vi "ChangeConfigServer.vi"(4 "error in (no error)":errorcluster) -> (0 "error out":errorcluster)   [LabVIEW 2015]
doc: "This GUI interprets supplied configuration information and displays it to the user. It compares the target configuration to the machine state (what components are loaded) and checks for compatibility. If the user choses to start a move, an enumerated script is output that can be used to start a sequence of moves."
uses:
  Script_actions.ctl
  Utils/ChangeConfig.ctl
  Users/Sherman/Desktop/BETA_GSCS/Systems/SystemUtil/Command.ctl
  Users/Sherman/Desktop/BETA_GSCS/GUI/GSP_GUI_global.vi
  TCPServer/TCP_Global.vi
panel:
  out "First Attempt to change?":bool
  out "Used setup Cmd":bool
  in  "Configuration":i32(listbox)
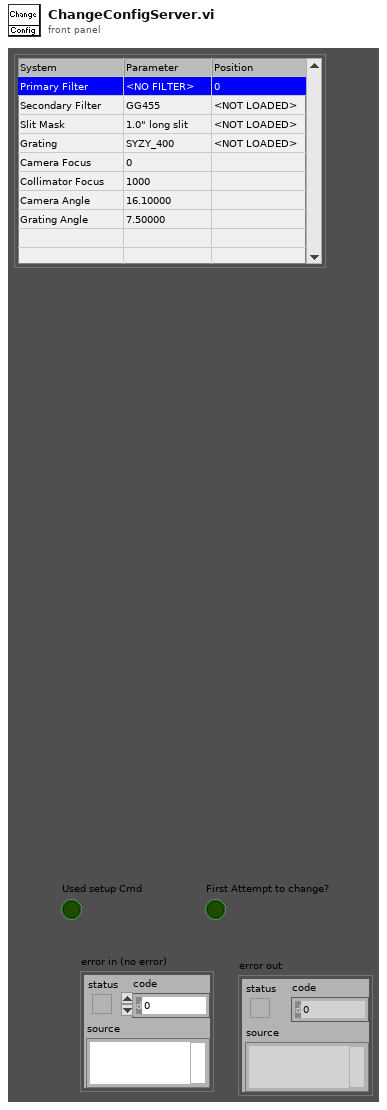
[diagram p1: front panel]
types:
  T1 = typedef "Command.ctl" = cluster{"Command":string, "Parameter":string}
  T2 = typedef "ChangeConfig.ctl" = cluster{"Command":string, "Configuration":cluster{"Primary Filter":string, "Secondary Filter":string, "Slit Mask":string, "Grating":string, "CS Target":dbl, "GS Target":dbl, "Coll Focus":i32, "Camera Focus":i32, "use Flexure Comp?":bool, "WavMode":string, "Slit Toggle":string}}
  T3 = cluster{"Primary Filter Slot":i32, "Secondary Filter Slot":i32, "Slit#":i32, "Grating#":i32, "CS Angle":dbl, "GS Angle":dbl, "Coll Focus":i32, "Camera Focus":i32, "Select Mode":i32, "Flexure":bool, "Slit Toggle":bool}
  T4 = typedef "Script_actions.ctl" = enum16{"Change Primary Filter", "Change Secondary Filter", "Change Collimator Focus", "Change Camera Focus", "Change Grating", "Change Angles", "Change Slit Mask", "Toggle Slit", "Change WAVMODE", "Check All Systems", "Change Flexure"}
  T5 = cluster{"Grating#":i32, "Slit#":i32, "Primary Filter#":i32, "Secondary Filter#":i32, "Coll Position":i32, "Camera Focus":i32, "Camera Angle":dbl, "Grating Angle":dbl, "Coll Temp":dbl, "CF Temp\n":dbl, "Camera Target":dbl, "Grating Target":dbl, "WAVMODE":string, "Slit Hidden??":bool}
  T6 = cluster{"Primary Filter":string, "Secondary Filter":string, "Slit Mask":string, "Grating":string, "CS Target":dbl, "GS Target":dbl, "Coll Focus":i32, "Camera Focus":i32, "use Flexure Comp?":bool, "WavMode":string, "Slit Toggle":string}
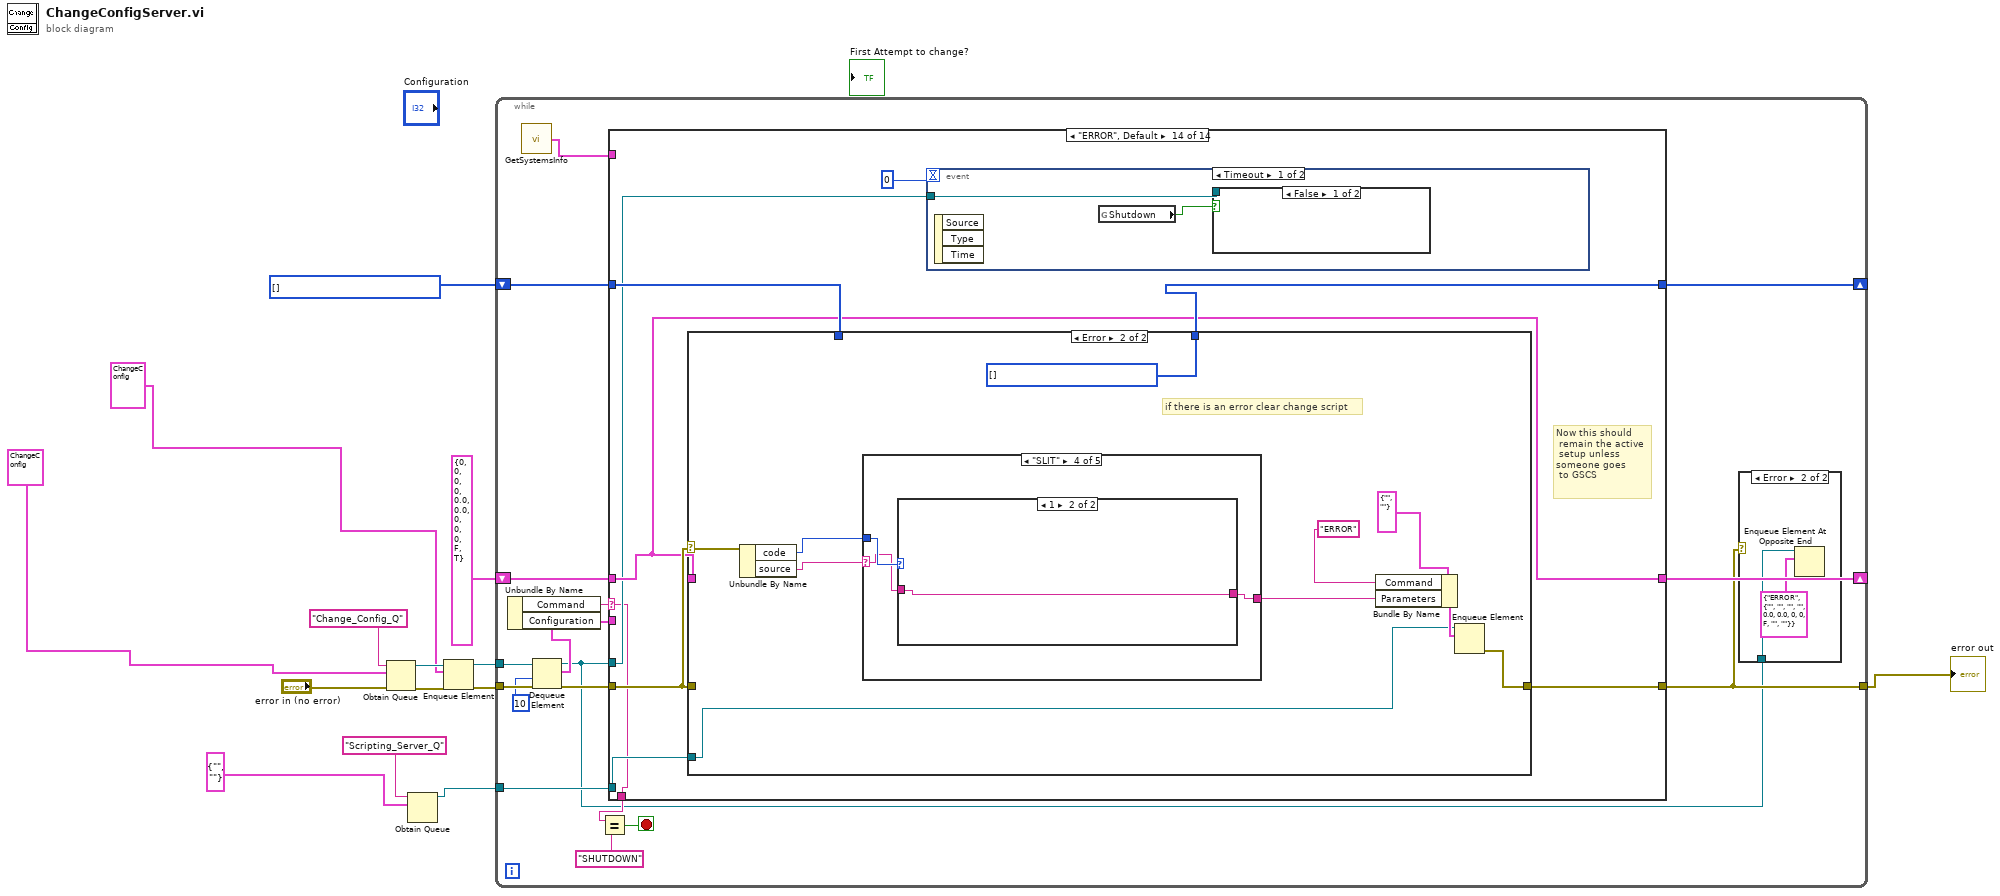
[diagram p0: block diagram]
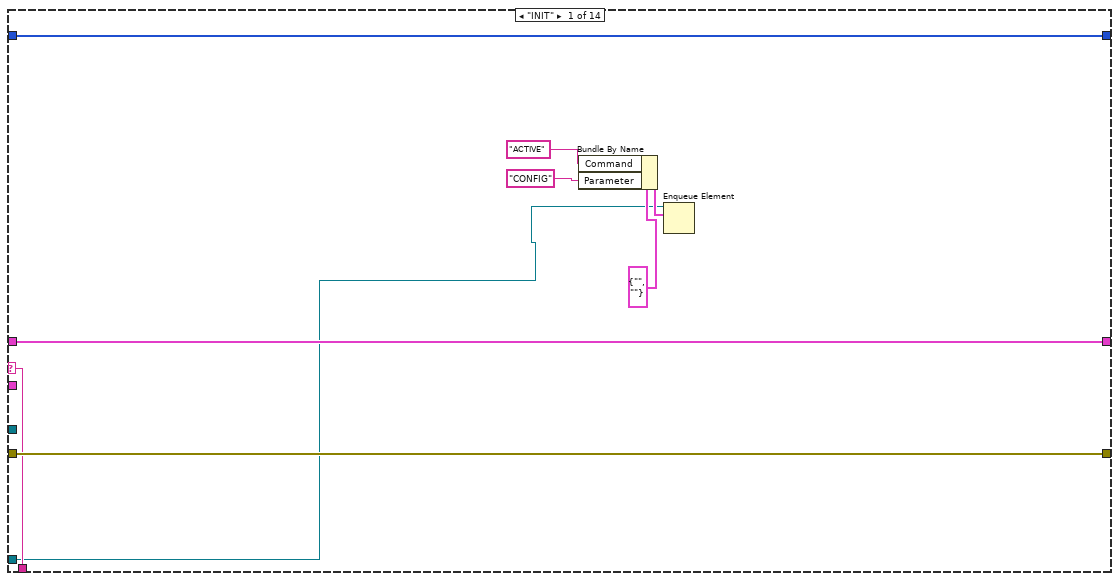
[diagram p3: hidden frame]
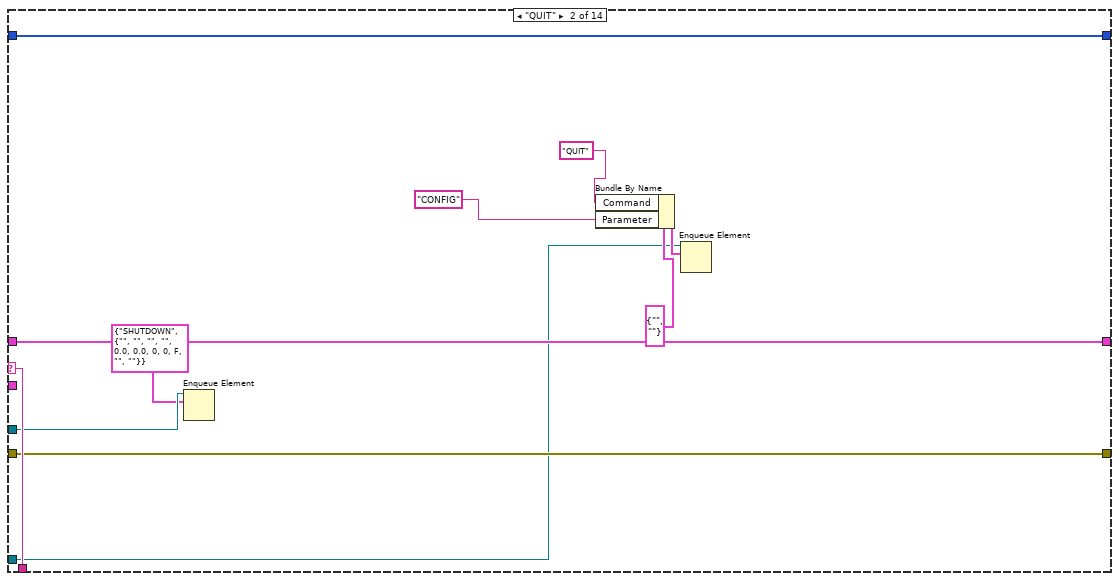
[diagram p4: hidden frame]
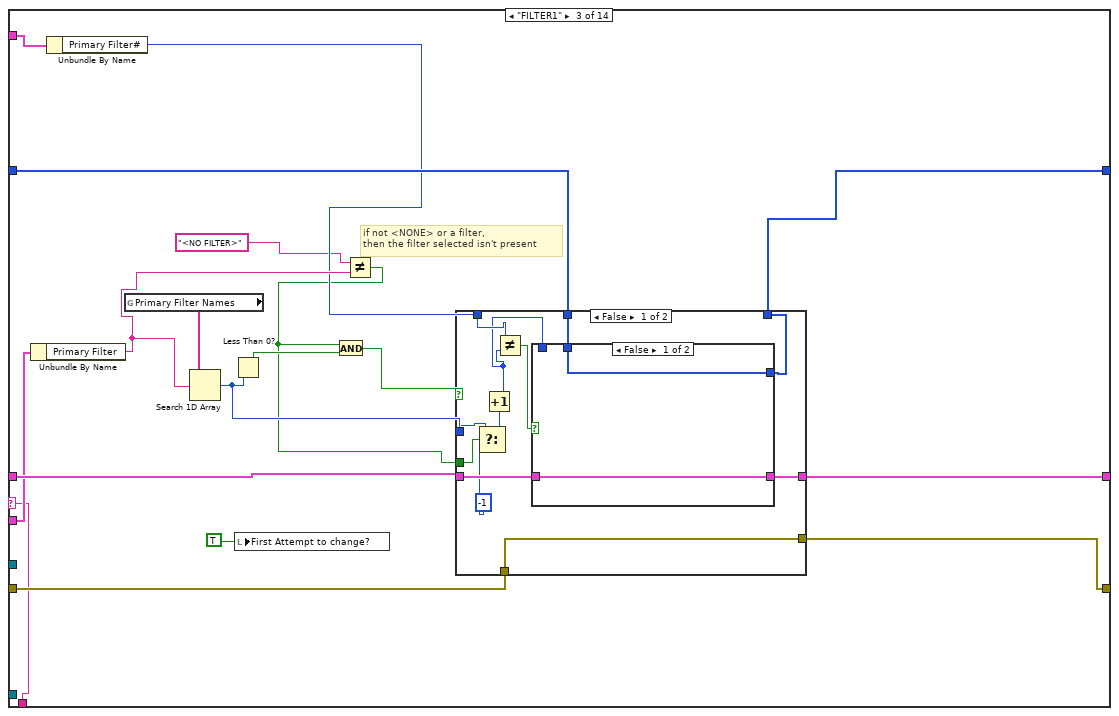
[diagram p5: hidden frame]
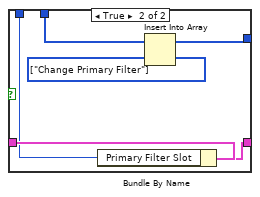
[diagram p6: hidden frame]
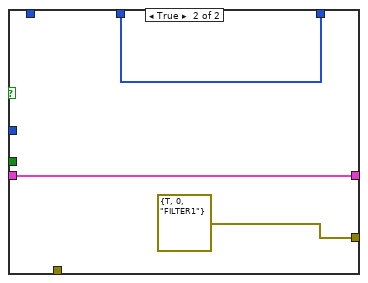
[diagram p7: hidden frame]
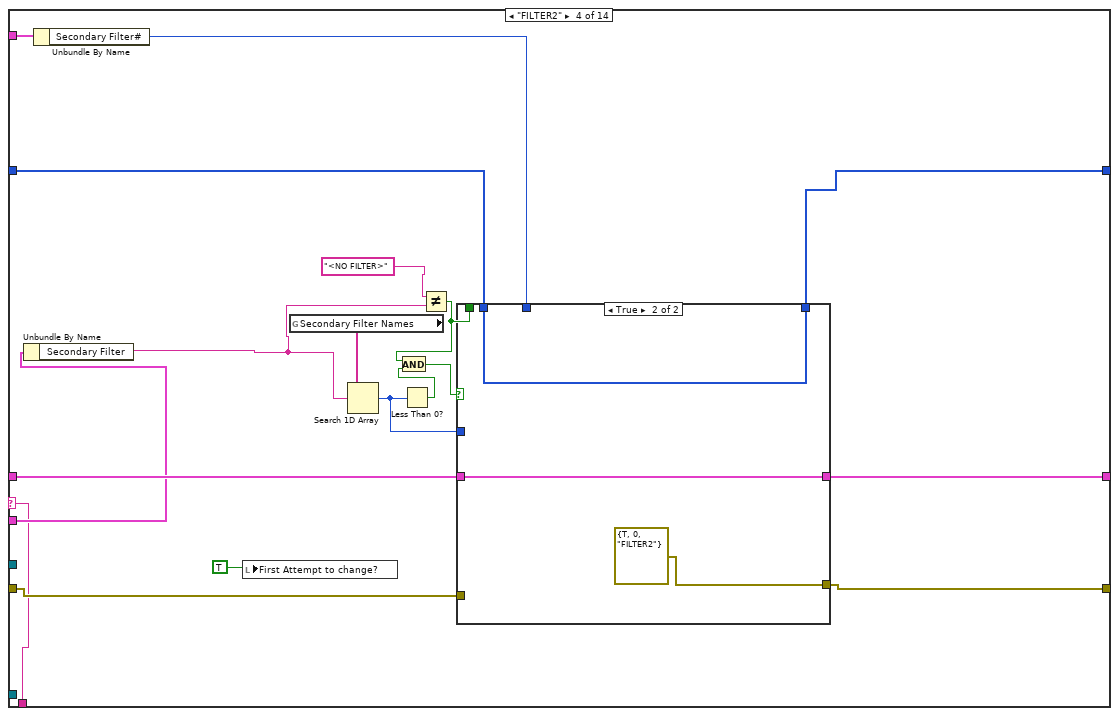
[diagram p8: hidden frame]
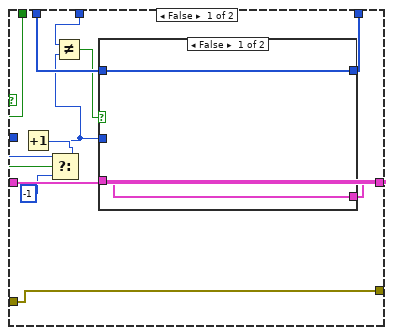
[diagram p9: hidden frame]
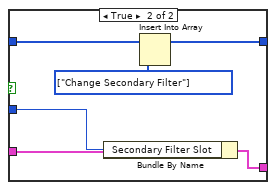
[diagram p10: hidden frame]
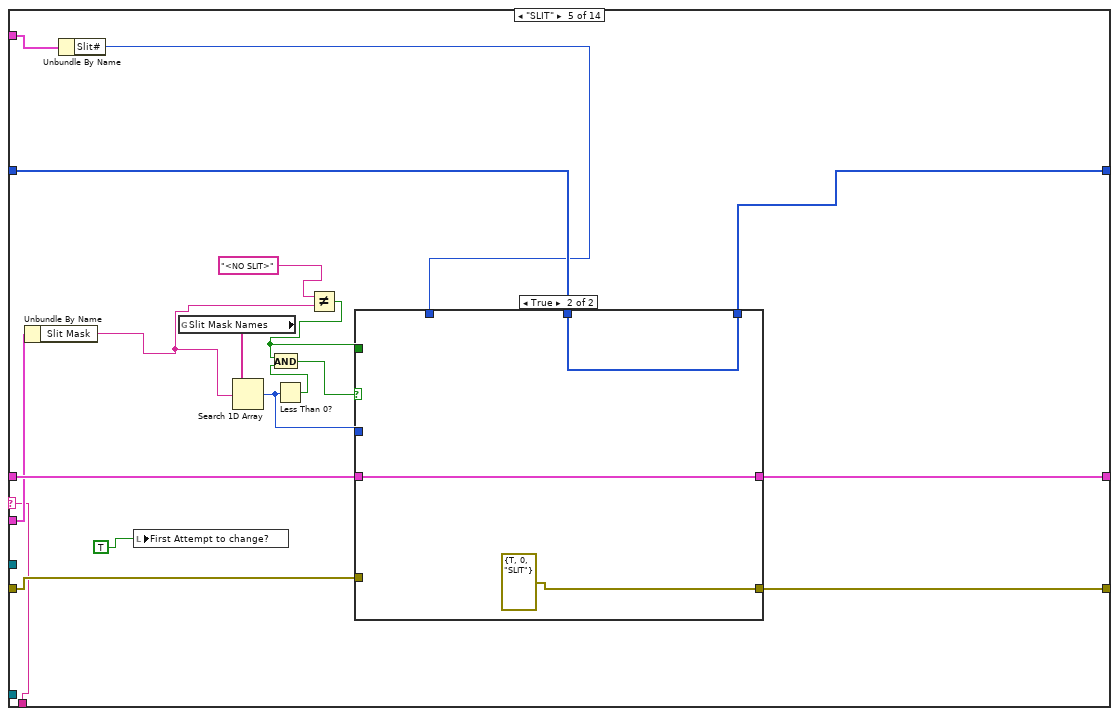
[diagram p11: hidden frame]
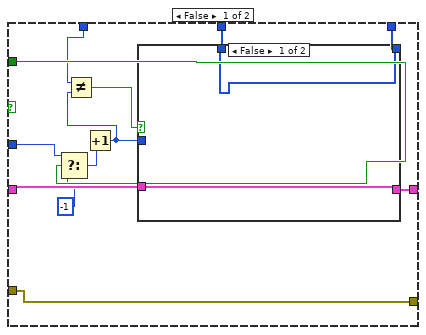
[diagram p12: hidden frame]
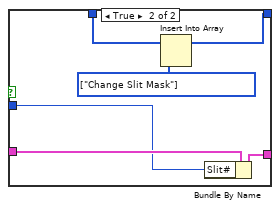
[diagram p13: hidden frame]
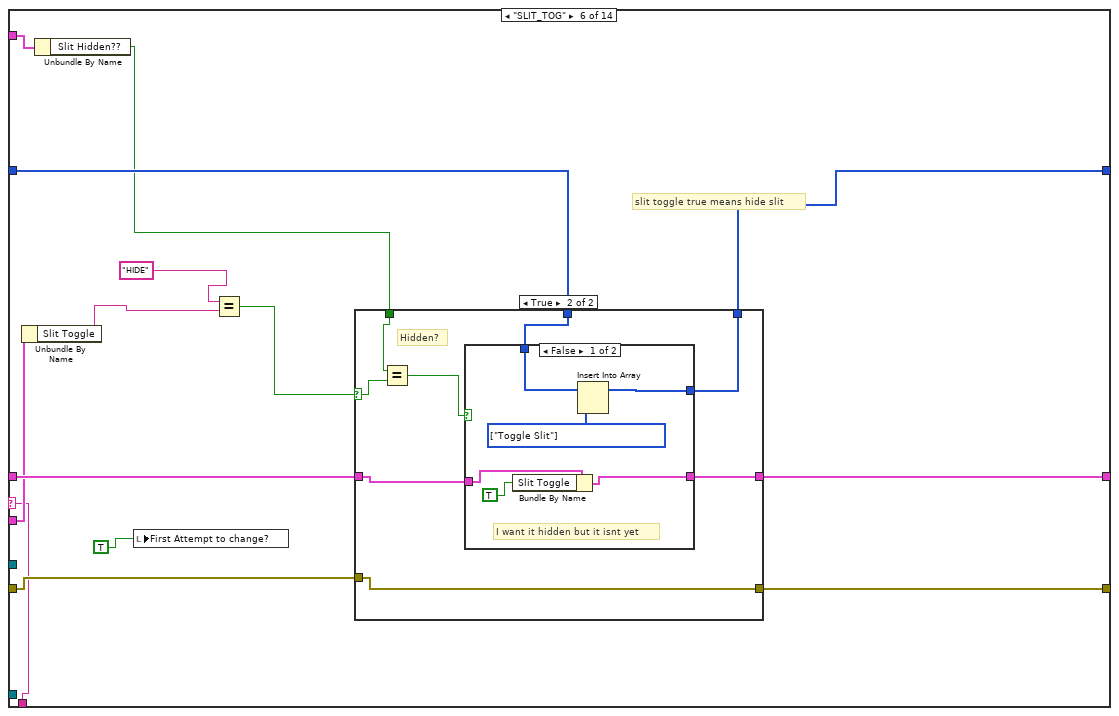
[diagram p14: hidden frame]
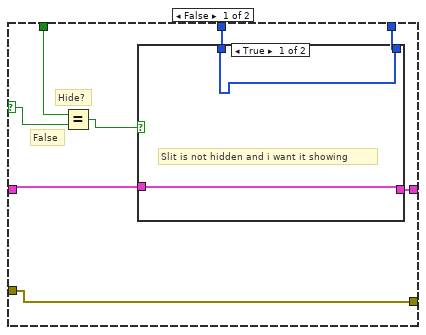
[diagram p15: hidden frame]
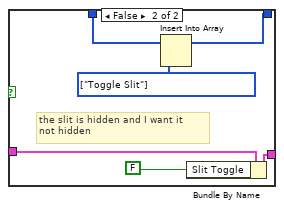
[diagram p16: hidden frame]
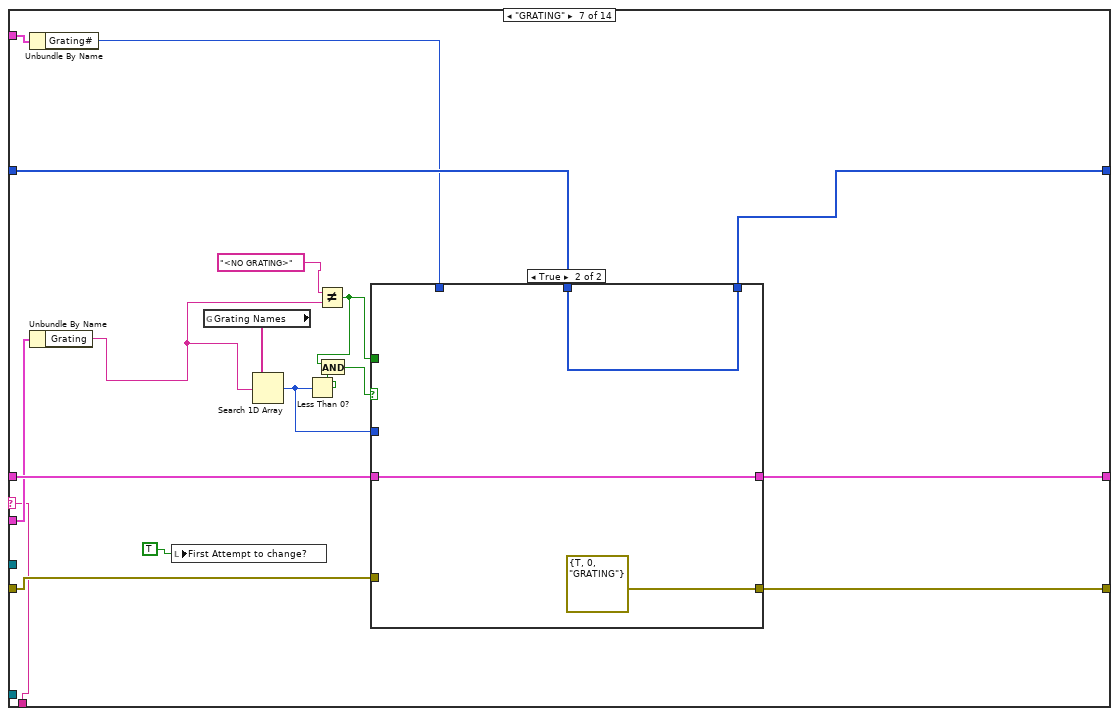
[diagram p18: hidden frame]
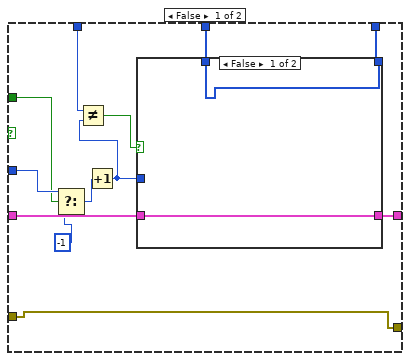
[diagram p19: hidden frame]
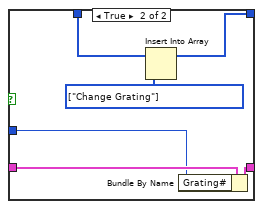
[diagram p20: hidden frame]
diagram:
  w8 = T4[] [] items=["Change Primary Filter", "Change Secondary Filter", "Change Collimator Focus", "Change Camera Focus", "Change Grating", "Change Angles", "Change Slit Mask", "Toggle Slit", "Change WAVMODE", "Check All Systems", "Change Flexure"]
  n1 = Obtain Queue(name (unnamed)="Change_Config_Q", element data type=T2 {"Command"="", "Configuration"={"Primary Filter"="", "Secondary Filter"="", "Slit Mask"="", "Grating"="", "CS Target"=0.0, "GS Target"=0.0, "Coll Focus"=0, "Camera Focus"=0, "use Flexure Comp?"=FALSE, "WavMode"="", "Slit Toggle"=""}} ("Cluster"), error in (no error)="error in (no error)") -> (queue out=w10:refnum<queue>, error out=w11:errorcluster)  [unwired: 2 in, 1 out]
  n2 = Obtain Queue(name (unnamed)="Scripting_Server_Q", element data type=T1 {"Command"="", "Parameter"=""} ("Command")) -> (queue out=w2:refnum<queue>)  [unwired: 3 in, 2 out]
  n3 = Enqueue Element(queue=w10, element=T2 {"Command"="INIT", "Configuration"={"Primary Filter"="", "Secondary Filter"="", "Slit Mask"="", "Grating"="", "CS Target"=0.0, "GS Target"=0.0, "Coll Focus"=0, "Camera Focus"=0, "use Flexure Comp?"=FALSE, "WavMode"="", "Slit Toggle"=""}} ("Cluster"), error in (no error)=w11) -> (queue out=w9:refnum<queue>, error out=w12:errorcluster)  [unwired: 1 in, 1 out]
  n4 = while {
    tunnel: w12 -> [w32]
    tunnel: [w16] -> w4
    tunnel: w9 -> [w30]
    shift-right: [w25] -> _
    shift-left: w8 -> [w26]
    shift-right: [w23] -> _
    shift-left: T3 {"Primary Filter Slot"=0, "Secondary Filter Slot"=0, "Slit#"=0, "Grating#"=0, "CS Angle"=0.0, "GS Angle"=0.0, "Coll Focus"=0, "Camera Focus"=0, "Select Mode"=0, "Flexure"=FALSE, "Slit Toggle"=TRUE} ("Targets") -> [w24]
    tunnel: w2 -> [w18]
    stop <- w28 stop-if-true
    n5 = call "GetSystemsInfo.vi"() -> ("Pos Info"=w22:T5)
    n6 = Dequeue Element(queue=w30, timeout in ms (-1)=10, error in (no error)=w32) -> (queue out=w15:refnum<queue>, element=w21:T2, error out=w31:errorcluster)  [unwired: 1 out]
    n7 = Unbundle By Name(w21) -> ("Command"=w20:string, "Configuration"=w19:T6)
    n8 = case shown="\"ERROR\", Default" w20 {
      selector: w20 -> [w40 w54 w55 w96 w137 w178 w224 w265 w291 w322 w348 w366 w378 w395]
      tunnel: w31 -> [w42 w53 w58 w99 w140 w184 w227 w274 w305 w336 w359 w368 w382 w400]
      tunnel: [w42 w53 w57 w98 w139 w183 w226 w273 w304 w336 w359 w368 w376 w403] -> w16
      tunnel: w15 -> [_ w45 _ _ _ _ _ _ _ _ _ _ w385 w396]
      tunnel: w26 -> [w43 w51 w71 w112 w154 w191 w241 w280 w311 w341 w361 w374 w381 w401]
      tunnel: [w43 w51 w70 w111 w153 w190 w240 w279 w310 w340 w360 w373 w381 w399] -> w25
      tunnel: w24 -> [w41 w52 w69 w110 w152 w189 w239 w278 w309 w343 w358 w372 w380 w398]
      tunnel: [w41 w52 w68 w109 w151 w188 w238 w277 w308 w342 w357 w369 w380 w398] -> w23
      tunnel: w22 -> [_ _ w67 w108 w150 w187 w237 w276 w307 w339 w356 _ _ _]
      tunnel: w19 -> [_ _ w65 w106 w147 w186 w235 w275 w306 w337 w353 w371 w384 _]
      tunnel: w18 -> [w35 w46 _ _ _ _ _ _ _ _ _ _ _ w402]
      tunnel: [w40 w54 w55 w96 w137 w178 w224 w265 w291 w322 w348 w366 w378 w395] -> w17
      frame "INIT" {
        n9 = Bundle By Name(cluster=T1 {"Command"="", "Parameter"=""} ("Command"), "Command"="ACTIVE", "Parameter"="CONFIG") -> (w37:T1)
        n10 = Enqueue Element(queue=w35, element=w37) -> ()  [unwired: 2 in, 3 out]
      }
      frame "QUIT" {
        n11 = Enqueue Element(queue=w45, element=T2 {"Command"="SHUTDOWN", "Configuration"={"Primary Filter"="", "Secondary Filter"="", "Slit Mask"="", "Grating"="", "CS Target"=0.0, "GS Target"=0.0, "Coll Focus"=0, "Camera Focus"=0, "use Flexure Comp?"=FALSE, "WavMode"="", "Slit Toggle"=""}} ("Cluster")) -> ()  [unwired: 2 in, 3 out]
        n12 = Bundle By Name(cluster=T1 {"Command"="", "Parameter"=""} ("Command"), "Command"="QUIT", "Parameter"="CONFIG") -> (w48:T1)
        n13 = Enqueue Element(queue=w46, element=w48) -> ()  [unwired: 2 in, 3 out]
      }
      frame "FILTER1" {
        # "if not <NONE> or a filter, \nthen the filter selected isn't present"
        n14 = Unbundle By Name(w65) -> ("Primary Filter"=w72:string)
        n15 = Unbundle By Name(w67) -> ("Primary Filter#"=w66:i32)
        n16 = global read "GSP_GUI_global.vi" "Primary Filter Names"() -> (w64:string[])
        n17 = Search 1D Array(1D array=w64, element=w72) -> (index of element=w63:i32)  [unwired: 1 in]
        n18 = Less Than 0?(x=w63) -> (x < 0?=w61:bool)
        n19 = local write "First Attempt to change?"(TRUE) -> ()
        n20 = Not Equal?(x="<NO FILTER>", y=w72) -> (x != y?=w59:bool)
        n21 = And(x=w59, y=w61) -> (x .and. y?=w60:bool)
        n22 = case shown="False" w60 {
          tunnel: w63 -> [w79 _]
          tunnel: w71 -> [w84 w95]
          tunnel: [w83 w95] -> w70
          tunnel: w69 -> [w82 w94]
          tunnel: [w81 w94] -> w68
          tunnel: w59 -> [w77 _]
          tunnel: w66 -> [w76 _]
          tunnel: w58 -> [w73 _]
          tunnel: [w73 errorcluster {"status"=TRUE, "code"=0, "source"="FILTER1"} ("error constant")] -> w57
          frame False {
            n23 = Select(t=w79, s=w77, f=-1) -> (s? t:f=w78:i32)
            n24 = Increment(x=w78) -> (x+1=w74:i32)
            n25 = Not Equal?(x=w76, y=w74) -> (x != y?=w75:bool)
            n26 = case shown="False" w75 {
              tunnel: w84 -> [w86 w92]
              tunnel: [w86 w91] -> w83
              tunnel: w82 -> [w85 w90]
              tunnel: [w85 w89] -> w81
              tunnel: w74 -> [_ w88]
              frame False {
              }
              frame True {
                w87 = T4[] [enum."Change Primary Filter"] items=["Change Primary Filter", "Change Secondary Filter", "Change Collimator Focus", "Change Camera Focus", "Change Grating", "Change Angles", "Change Slit Mask", "Toggle Slit", "Change WAVMODE", "Check All Systems", "Change Flexure"]
                n27 = Bundle By Name(cluster=w90, "Primary Filter Slot"=w88) -> (w89:T3)
                n28 = Insert Into Array(array=w92, new element=w87) -> (w91:T4[])  [unwired: 1 in]
              }
            }
          }
          frame True {
          }
        }
      }
      frame "FILTER2" {
        n29 = Unbundle By Name(w106) -> ("Secondary Filter"=w113:string)
        n30 = Unbundle By Name(w108) -> ("Secondary Filter#"=w107:i32)
        n31 = local write "First Attempt to change?"(TRUE) -> ()
        n32 = global read "GSP_GUI_global.vi" "Secondary Filter Names"() -> (w105:string[])
        n33 = Search 1D Array(1D array=w105, element=w113) -> (index of element=w104:i32)  [unwired: 1 in]
        n34 = Less Than 0?(x=w104) -> (x < 0?=w102:bool)
        n35 = Not Equal?(x="<NO FILTER>", y=w113) -> (x != y?=w100:bool)
        n36 = And(x=w100, y=w102) -> (x .and. y?=w101:bool)
        n37 = case shown="True" w101 {
          tunnel: w104 -> [w120 _]
          tunnel: w112 -> [w125 w136]
          tunnel: [w124 w136] -> w111
          tunnel: w110 -> [w123 w135]
          tunnel: [w122 w135] -> w109
          tunnel: w100 -> [w118 _]
          tunnel: w107 -> [w117 _]
          tunnel: w99 -> [w114 _]
          tunnel: [w114 errorcluster {"status"=TRUE, "code"=0, "source"="FILTER2"} ("error constant")] -> w98
          frame False {
            n38 = Select(t=w120, s=w118, f=-1) -> (s? t:f=w119:i32)
            n39 = Increment(x=w119) -> (x+1=w116:i32)
            n40 = Not Equal?(x=w117, y=w116) -> (x != y?=w115:bool)
            n41 = case shown="False" w115 {
              tunnel: w125 -> [w126 w133]
              tunnel: [w126 w132] -> w124
              tunnel: w123 -> [w127 w131]
              tunnel: [w127 w130] -> w122
              tunnel: w116 -> [_ w129]
              frame False {
              }
              frame True {
                w128 = T4[] [enum."Change Secondary Filter"] items=["Change Primary Filter", "Change Secondary Filter", "Change Collimator Focus", "Change Camera Focus", "Change Grating", "Change Angles", "Change Slit Mask", "Toggle Slit", "Change WAVMODE", "Check All Systems", "Change Flexure"]
                n42 = Bundle By Name(cluster=w131, "Secondary Filter Slot"=w129) -> (w130:T3)
                n43 = Insert Into Array(array=w133, new element=w128) -> (w132:T4[])  [unwired: 1 in]
              }
            }
          }
          frame True {
          }
        }
      }
      frame "SLIT" {
        n44 = Unbundle By Name(w147) -> ("Slit Mask"=w148:string)
        n45 = Unbundle By Name(w150) -> ("Slit#"=w149:i32)
        n46 = local write "First Attempt to change?"(TRUE) -> ()
        n47 = global read "GSP_GUI_global.vi" "Slit Mask Names"() -> (w146:string[])
        n48 = Search 1D Array(1D array=w146, element=w148) -> (index of element=w145:i32)  [unwired: 1 in]
        n49 = Less Than 0?(x=w145) -> (x < 0?=w143:bool)
        n50 = Not Equal?(x="<NO SLIT>", y=w148) -> (x != y?=w141:bool)
        n51 = And(x=w141, y=w143) -> (x .and. y?=w142:bool)
        n52 = case shown="True" w142 {
          tunnel: w145 -> [w162 _]
          tunnel: w154 -> [w166 w177]
          tunnel: [w165 w177] -> w153
          tunnel: w152 -> [w164 w176]
          tunnel: [w163 w176] -> w151
          tunnel: w141 -> [w161 _]
          tunnel: w149 -> [w157 _]
          tunnel: w140 -> [w155 _]
          tunnel: [w155 errorcluster {"status"=TRUE, "code"=0, "source"="SLIT"} ("error constant")] -> w139
          frame False {
            n53 = Select(t=w162, s=w161, f=-1) -> (s? t:f=w159:i32)
            n54 = Increment(x=w159) -> (x+1=w158:i32)
            n55 = Not Equal?(x=w157, y=w158) -> (x != y?=w156:bool)
            n56 = case shown="False" w156 {
              tunnel: w166 -> [w167 w174]
              tunnel: [w167 w173] -> w165
              tunnel: w164 -> [w168 w172]
              tunnel: [w168 w171] -> w163
              tunnel: w158 -> [_ w170]
              frame False {
              }
              frame True {
                w169 = T4[] [enum."Change Slit Mask"] items=["Change Primary Filter", "Change Secondary Filter", "Change Collimator Focus", "Change Camera Focus", "Change Grating", "Change Angles", "Change Slit Mask", "Toggle Slit", "Change WAVMODE", "Check All Systems", "Change Flexure"]
                n57 = Insert Into Array(array=w174, new element=w169) -> (w173:T4[])  [unwired: 1 in]
                n58 = Bundle By Name(cluster=w172, "Slit#"=w170) -> (w171:T3)
              }
            }
          }
          frame True {
          }
        }
      }
      frame "SLIT_TOG" {
        # "slit toggle true means hide slit"
        n59 = Unbundle By Name(w186) -> ("Slit Toggle"=w181:string)
        n60 = Unbundle By Name(w187) -> ("Slit Hidden??"=w179:bool)
        n61 = local write "First Attempt to change?"(TRUE) -> ()
        n62 = Equal?(x="HIDE", y=w181) -> (x = y?=w180:bool)
        n63 = case shown="True" w180 {
          selector: w180 -> [w193 w214]
          tunnel: w191 -> [w199 w209]
          tunnel: [w198 w208] -> w190
          tunnel: w189 -> [w197 w211]
          tunnel: [w196 w210] -> w188
          tunnel: w184 -> [w195 w213]
          tunnel: [w195 w213] -> w183
          tunnel: w179 -> [w194 w215]
          frame False {
            # "Hide?"
            # "False"
            n64 = Equal?(x=w194, y=w193) -> (x = y?=w192:bool)
            n65 = case shown="True" w192 {
              tunnel: w199 -> [w200 w207]
              tunnel: [w200 w206] -> w198
              tunnel: w197 -> [w201 w205]
              tunnel: [w201 w204] -> w196
              frame True {
                # "Slit is not hidden and i want it showing"
              }
              frame False {
                w203 = T4[] [enum."Toggle Slit"] items=["Change Primary Filter", "Change Secondary Filter", "Change Collimator Focus", "Change Camera Focus", "Change Grating", "Change Angles", "Change Slit Mask", "Toggle Slit", "Change WAVMODE", "Check All Systems", "Change Flexure"]
                # "the slit is hidden and I want it \nnot hidden"
                n66 = Insert Into Array(array=w207, new element=w203) -> (w206:T4[])  [unwired: 1 in]
                n67 = Bundle By Name(cluster=w205, "Slit Toggle"=FALSE) -> (w204:T3)
              }
            }
          }
          frame True {
            # "Hidden?"
            n68 = Equal?(x=w215, y=w214) -> (x = y?=w212:bool)
            n69 = case shown="False" w212 {
              tunnel: w211 -> [w218 w223]
              tunnel: [w217 w223] -> w210
              tunnel: w209 -> [w220 w222]
              tunnel: [w219 w222] -> w208
              frame False {
                w221 = T4[] [enum."Toggle Slit"] items=["Change Primary Filter", "Change Secondary Filter", "Change Collimator Focus", "Change Camera Focus", "Change Grating", "Change Angles", "Change Slit Mask", "Toggle Slit", "Change WAVMODE", "Check All Systems", "Change Flexure"]
                # "I want it hidden but it isnt yet"
                n70 = Bundle By Name(cluster=w218, "Slit Toggle"=TRUE) -> (w217:T3)
                n71 = Insert Into Array(array=w220, new element=w221) -> (w219:T4[])  [unwired: 1 in]
              }
              frame True {
                # "I want it hidden and its hidden"
              }
            }
          }
        }
      }
      frame "GRATING" {
        n72 = Unbundle By Name(w237) -> ("Grating#"=w236:i32)
        n73 = Unbundle By Name(w235) -> ("Grating"=w234:string)
        n74 = local write "First Attempt to change?"(TRUE) -> ()
        n75 = global read "GSP_GUI_global.vi" "Grating Names"() -> (w233:string[])
        n76 = Search 1D Array(1D array=w233, element=w234) -> (index of element=w232:i32)  [unwired: 1 in]
        n77 = Less Than 0?(x=w232) -> (x < 0?=w231:bool)
        n78 = Not Equal?(x="<NO GRATING>", y=w234) -> (x != y?=w229:bool)
        n79 = And(x=w229, y=w231) -> (x .and. y?=w228:bool)
        n80 = case shown="True" w228 {
          tunnel: w232 -> [w248 _]
          tunnel: w241 -> [w253 w264]
          tunnel: [w252 w264] -> w240
          tunnel: w239 -> [w251 w263]
          tunnel: [w250 w263] -> w238
          tunnel: w229 -> [w246 _]
          tunnel: w236 -> [w243 _]
          tunnel: w227 -> [w242 _]
          tunnel: [w242 errorcluster {"status"=TRUE, "code"=0, "source"="GRATING"} ("error constant")] -> w226
          frame False {
            n81 = Select(t=w248, s=w246, f=-1) -> (s? t:f=w247:i32)
            n82 = Increment(x=w247) -> (x+1=w244:i32)
            n83 = Not Equal?(x=w243, y=w244) -> (x != y?=w245:bool)
            n84 = case shown="False" w245 {
              tunnel: w253 -> [w255 w261]
              tunnel: [w255 w260] -> w252
              tunnel: w251 -> [w254 w259]
              tunnel: [w254 w258] -> w250
              tunnel: w244 -> [_ w257]
              frame False {
              }
              frame True {
                w256 = T4[] [enum."Change Grating"] items=["Change Primary Filter", "Change Secondary Filter", "Change Collimator Focus", "Change Camera Focus", "Change Grating", "Change Angles", "Change Slit Mask", "Toggle Slit", "Change WAVMODE", "Check All Systems", "Change Flexure"]
                n85 = Insert Into Array(array=w261, new element=w256) -> (w260:T4[])  [unwired: 1 in]
                n86 = Bundle By Name(cluster=w259, "Grating#"=w257) -> (w258:T3)
              }
            }
          }
          frame True {
          }
        }
      }
      frame "COLL_FOCUS" {
        # "Check to make sure its in a good range"
        # "round"
        n87 = Unbundle By Name(w276) -> ("Coll Position"=w271:i32)
        n88 = Unbundle By Name(w275) -> ("Coll Focus"=w270:i32)
        n89 = local write "First Attempt to change?"(TRUE) -> ()
        n90 = Subtract(x=w271, y=w270) -> (x-y=w267:i32)
        n91 = Absolute Value(x=w267) -> (abs(x)=w266:i32)
        n92 = Greater?(x=w266, y=10) -> (0:w268:bool)
        n93 = case shown="True" w268 {
          tunnel: w280 -> [w283 w290]
          tunnel: [w283 w289] -> w279
          tunnel: w278 -> [w282 w288]
          tunnel: w270 -> [_ w287]
          tunnel: [w282 w286] -> w277
          tunnel: w274 -> [w281 w284]
          tunnel: [w281 w284] -> w273
          frame False {
            # "add not in range error"
          }
          frame True {
            w285 = T4[] [enum."Change Collimator Focus"] items=["Change Primary Filter", "Change Secondary Filter", "Change Collimator Focus", "Change Camera Focus", "Change Grating", "Change Angles", "Change Slit Mask", "Toggle Slit", "Change WAVMODE", "Check All Systems", "Change Flexure"]
            n94 = Bundle By Name(cluster=w288, "Coll Focus"=w287) -> (w286:T3)
            n95 = Insert Into Array(array=w290, new element=w285) -> (w289:T4[])  [unwired: 1 in]
          }
        }
      }
      frame "CAMERA_FOCUS" {
        # "add not in range error"
        # "round"
        n96 = Unbundle By Name(w306) -> ("Camera Focus"=w299:i32)
        n97 = Unbundle By Name(w307) -> ("Camera Focus"=w296:i32)
        n98 = Square(x=w299) -> (x^2=w301:i32)
        n99 = Square Root(x=w301) -> (sqrt(x)=w298:dbl)
        n100 = local write "First Attempt to change?"(TRUE) -> ()
        n101 = Square(x=w296) -> (x^2=w297:i32)
        n102 = Square Root(x=w297) -> (sqrt(x)=w295:dbl)
        n103 = Subtract(x=w295, y=w298) -> (x-y=w293:dbl)
        n104 = Square(x=w293) -> (x^2=w294:dbl)
        n105 = Square Root(x=w294) -> (sqrt(x)=w292:dbl)
        n106 = Greater?(x=w292, y=10) -> (0:w302:bool)
        n107 = case shown="False" w302 {
          tunnel: w311 -> [w313 w321]
          tunnel: [w313 w320] -> w310
          tunnel: w309 -> [w314 w319]
          tunnel: w299 -> [_ w318]
          tunnel: [w314 w317] -> w308
          tunnel: w305 -> [w312 w315]
          tunnel: [w312 w315] -> w304
          frame False {
          }
          frame True {
            w316 = T4[] [enum."Change Camera Focus"] items=["Change Primary Filter", "Change Secondary Filter", "Change Collimator Focus", "Change Camera Focus", "Change Grating", "Change Angles", "Change Slit Mask", "Toggle Slit", "Change WAVMODE", "Check All Systems", "Change Flexure"]
            n108 = Bundle By Name(cluster=w319, "Camera Focus"=w318) -> (w317:T3)
            n109 = Insert Into Array(array=w321, new element=w316) -> (w320:T4[])  [unwired: 1 in]
          }
        }
      }
      frame "LOAD_DOUBLES" {
        # "maybe make error if the doubles arent going to make light?"
        # "round"
        n110 = Unbundle By Name(w339) -> ("Camera Angle"=w333:dbl, "Grating Angle"=w329:dbl)
        n111 = Unbundle By Name(w337) -> ("CS Target"=w332:dbl, "GS Target"=w330:dbl)
        n112 = Subtract(x=w333, y=w332) -> (x-y=w324:dbl)
        n113 = Subtract(x=w329, y=w330) -> (x-y=w326:dbl)
        n114 = Absolute Value(x=w326) -> (abs(x)=w325:dbl)
        n115 = Absolute Value(x=w324) -> (abs(x)=w323:dbl)
        n116 = Greater?(x=w325, y=0.5) -> (0:w327:bool)
        n117 = Greater?(x=w323, y=0.5) -> (0:w331:bool)
        n118 = Bundle By Name(cluster=w343, "CS Angle"=w332, "GS Angle"=w330) -> (w342:T3)
        n119 = local write "First Attempt to change?"(TRUE) -> ()
        n120 = Or(x=w331, y=w327) -> (x .or. y?=w338:bool)
        n121 = case shown="True" w338 {
          tunnel: w341 -> [w344 w347]
          tunnel: [w344 w346] -> w340
          frame False {
          }
          frame True {
            w345 = T4[] [enum."Change Angles"] items=["Change Primary Filter", "Change Secondary Filter", "Change Collimator Focus", "Change Camera Focus", "Change Grating", "Change Angles", "Change Slit Mask", "Toggle Slit", "Change WAVMODE", "Check All Systems", "Change Flexure"]
            n122 = Insert Into Array(array=w347, new element=w345) -> (w346:T4[])  [unwired: 1 in]
          }
        }
      }
      frame "WAVMODE" {
        # "what if not equal but not in mode names?"
        # "Compare Wavemodes"
        n123 = Unbundle By Name(w356) -> ("WAVMODE"=w355:string)
        n124 = Unbundle By Name(w353) -> ("WavMode"=w351:string)
        n125 = global read "GSP_GUI_global.vi" "Standard Observing Mode Names"() -> (w352:string[])
        n126 = Not Equal?(x=w355, y=w351) -> (x != y?=w354:bool)
        n127 = Search 1D Array(1D array=w352, element=w351) -> (index of element=w350:i32)  [unwired: 1 in]
        n128 = Bundle By Name(cluster=w358, "Select Mode"=w350) -> (w357:T3)
        n129 = case shown="True" w354 {
          tunnel: w361 -> [w362 w365]
          tunnel: [w362 w364] -> w360
          frame False {
          }
          frame True {
            w363 = T4[] [enum."Change WAVMODE"] items=["Change Primary Filter", "Change Secondary Filter", "Change Collimator Focus", "Change Camera Focus", "Change Grating", "Change Angles", "Change Slit Mask", "Toggle Slit", "Change WAVMODE", "Check All Systems", "Change Flexure"]
            n130 = Insert Into Array(array=w365, new element=w363) -> (w364:T4[])  [unwired: 1 in]
          }
        }
        n131 = local write "First Attempt to change?"(TRUE) -> ()
      }
      frame "FLEXURE" {
        w375 = T4[] [enum."Change Flexure"] items=["Change Primary Filter", "Change Secondary Filter", "Change Collimator Focus", "Change Camera Focus", "Change Grating", "Change Angles", "Change Slit Mask", "Toggle Slit", "Change WAVMODE", "Check All Systems", "Change Flexure"]
        # "honestly dont see how this can be wrong"
        n132 = Unbundle By Name(w371) -> ("use Flexure Comp?"=w370:bool)
        n133 = local write "First Attempt to change?"(TRUE) -> ()
        n134 = Bundle By Name(cluster=w372, "Flexure"=w370) -> (w369:T3)
        n135 = Insert Into Array(array=w374, new element=w375) -> (w373:T4[])  [unwired: 1 in]
      }
      frame "SETUP" {
        w379 = TRUE
        # "time delay to give scripting chance to \nsend change Si command\nbefore this is done"
        n136 = for {
          shift-right: [w393] -> w377
          shift-left: w382 -> [w394]
          tunnel: [w391] -> _
          tunnel: w385 -> [w390]
          tunnel: string[] ["FILTER1", "FILTER2", "SLIT", "GRATING", "LOAD_DOUBLES", "CAMERA_FOCUS", "COLL_FOCUS", "WAVMODE", "FLEXURE"] -> [w389] mode=indexing
          tunnel: w384 -> [w387]
          n137 = Bundle By Name(cluster=T2 {"Command"="", "Configuration"={"Primary Filter"="", "Secondary Filter"="", "Slit Mask"="", "Grating"="", "CS Target"=0.0, "GS Target"=0.0, "Coll Focus"=0, "Camera Focus"=0, "use Flexure Comp?"=FALSE, "WavMode"="", "Slit Toggle"=""}} ("Cluster"), "Command"=w389, "Configuration"=w387) -> (w386:T2)
          n138 = Enqueue Element(queue=w390, element=w386, timeout in ms (-1)=0 ("ms timeout (-1)"), error in (no error)=w394) -> (queue out=w391:refnum<queue>, error out=w393:errorcluster)  [unwired: 1 out]
        }
        n139 = local write "First Attempt to change?"(w379) -> ()
        n140 = call "Time Delay"("error in (no error)"=w377) -> ("error out"=w376:errorcluster)  [unwired: 10 in]
        "Used setup Cmd" <- w379
      }
      frame "ERROR", Default {
        # "Now this should\n remain the active\n setup unless\nsomeone goes\n to GSCS"
        n141 = case shown="Error" w400 {
          selector: w400 -> [_ w468]
          tunnel: w400 -> [w418 _]
          tunnel: [w411 w462] -> w403
          tunnel: w402 -> [w412 w463]
          tunnel: w398 -> [w417 _]
          tunnel: w401 -> [w416 _]
          tunnel: [w413 w459] -> w399
          frame No Error {
            w413 = T4[] [] items=["Change Primary Filter", "Change Secondary Filter", "Change Collimator Focus", "Change Camera Focus", "Change Grating", "Change Angles", "Change Slit Mask", "Toggle Slit", "Change WAVMODE", "Check All Systems", "Change Flexure"]
            # "if no error, go ahead and make"
            # "If change script isn't empty\n, make changes"
            n142 = local read "First Attempt to change?"() -> (w410:bool)
            n143 = Array Size(array=w416) -> (size(s)=w415:i32)
            n144 = Greater Than 0?(x=w415) -> (x > 0?=w414:bool)
            n145 = case shown="False" w414 {
              tunnel: w418 -> [w421 w438]
              tunnel: [w421 w431] -> w411
              tunnel: w416 -> [_ w437]
              tunnel: w417 -> [_ w436]
              tunnel: w412 -> [w419 w434]
              tunnel: w410 -> [w420 _]
              frame False {
                # "empty change script"
                n146 = case shown="False" w420 {
                  tunnel: w419 -> [_ w424]
                  frame False {
                    # "not first attempt. Set used setup cmd? to false since we've enteres the deafult loop\nwhile waiting for another command"
                    n147 = local write "Used setup Cmd"(FALSE) -> ()
                  }
                  frame True {
                    # "If a commad is called then first attempt goes to true. It is possible to call commands \nand have no change needed. In this case done command is still needed."
                    n148 = local write "First Attempt to change?"(FALSE) -> ()
                    n149 = Bundle By Name(cluster=cluster{"Command":string, "Parameters":string} {"Command"="", "Parameters"=""}, "Command"="DONE", "Parameters"="SETUPNOCHANGE") -> (w427:cluster{"Command":string, "Parameters":string})
                    n150 = Enqueue Element(queue=w424, element=w427) -> ()  [unwired: 2 in, 3 out]
                  }
                }
              }
              frame True {
                # "Change script has stuff"
                n151 = local write "First Attempt to change?"(FALSE) -> ()
                n152 = local read "Used setup Cmd"() -> (w430:bool)
                n153 = call "ChangeSetup.vi"("error in"=w438, "Targets"=w436, "Script"=w437) -> ("error out"=w435:errorcluster, "Done"=w433:string)  [unwired: 7 in]
                n154 = case shown="No Error" w435 {
                  selector: w435 -> [_ w458]
                  tunnel: [w447 w457] -> w431
                  tunnel: w433 -> [w442 w455]
                  tunnel: cluster{"Command":string, "Parameters":string} {"Command"="", "Parameters"=""} -> [w445 w448]
                  tunnel: w434 -> [w444 w450]
                  tunnel: w430 -> [w441 _]
                  frame No Error {
                    # "if you used setup command return that"
                    n155 = Select(t="SETUP", s=w441, f=w442) -> (s? t:f=w439:string)
                    n156 = Bundle By Name(cluster=w445, "Command"="DONE", "Parameters"=w439) -> (w446:cluster{"Command":string, "Parameters":string})
                    n157 = Enqueue Element(queue=w444, element=w446) -> (error out=w447:errorcluster)  [unwired: 2 in, 2 out]
                  }
                  frame Error {
                    n158 = Unbundle By Name(w458) -> ("code"=w454:i32, "source"=w452:string)
                    n159 = Number To Decimal String(number=w454) -> (decimal integer string=w453:string)  [unwired: 1 in]
                    n160 = Concatenate Strings(w455, w453, w452) -> (w451:string)
                    n161 = Bundle By Name(cluster=w448, "Command"="ERROR", "Parameters"=w451) -> (w449:cluster{"Command":string, "Parameters":string})
                    n162 = Enqueue Element(queue=w450, element=w449) -> (error out=w457:errorcluster)  [unwired: 2 in, 2 out]
                  }
                }
              }
            }
          }
          frame Error {
            w459 = T4[] [] items=["Change Primary Filter", "Change Secondary Filter", "Change Collimator Focus", "Change Camera Focus", "Change Grating", "Change Angles", "Change Slit Mask", "Toggle Slit", "Change WAVMODE", "Check All Systems", "Change Flexure"]
            # "if there is an error clear change script"
            n163 = Unbundle By Name(w468) -> ("code"=w466:i32, "source"=w467:string)
            n164 = case shown="\"SLIT\"" w467 {
              selector: w467 -> [w469 w472 w479 w487 w494]
              tunnel: w466 -> [_ w471 w478 w488 w496]
              tunnel: [w469 w470 w480 w486 w495] -> w460
              frame "", Default {
              }
              frame "FILTER1" {
                n165 = case shown="0, Default" w471 {
                  tunnel: w472 -> [w476 w477]
                  tunnel: [w473 w477] -> w470
                  frame 0, Default {
                    n166 = Concatenate Strings(w476, "NOT", "AVAILABLE") -> (w473:string)
                  }
                  frame 1 {
                  }
                }
              }
              frame "FILTER2" {
                n167 = case shown="0, Default" w478 {
                  tunnel: [w481 w485] -> w480
                  tunnel: w479 -> [w484 w485]
                  frame 0, Default {
                    n168 = Concatenate Strings(w484, "NOT", "AVAILABLE") -> (w481:string)
                  }
                  frame 1 {
                  }
                }
              }
              frame "SLIT" {
                n169 = case shown="1" w488 {
                  tunnel: [w489 w493] -> w486
                  tunnel: w487 -> [w492 w493]
                  frame 0, Default {
                    n170 = Concatenate Strings(w492, "NOT", "AVAILABLE") -> (w489:string)
                  }
                  frame 1 {
                  }
                }
              }
              frame "GRATING" {
                n171 = case shown="1" w496 {
                  tunnel: [w497 w501] -> w495
                  tunnel: w494 -> [w500 w501]
                  frame 0, Default {
                    n172 = Concatenate Strings(w500, "NOT", "AVAILABLE") -> (w497:string)
                  }
                  frame 1 {
                  }
                }
              }
            }
            n173 = Bundle By Name(cluster=cluster{"Command":string, "Parameters":string} {"Command"="", "Parameters"=""}, "Command"="ERROR", "Parameters"=w460) -> (w465:cluster{"Command":string, "Parameters":string})
            n174 = Enqueue Element(queue=w463, element=w465) -> (error out=w462:errorcluster)  [unwired: 2 in, 2 out]
          }
        }
        n175 = event shown="[0] Timeout" {
          selector: _ -> [_ _]
          dyn-events: _ -> [_ _]
          timeout: 0 -> [_ _]
          tunnel: w396 -> [w405 w408]
          event Timeout {
            n176 = event-data() -> ()  [unwired: 1 in, 3 out]
            n177 = global read "TCP_Global.vi" "Shutdown"() -> (w404:bool)
            n178 = case shown="False" w404 {
              tunnel: w405 -> [_ w406]
              frame False {
              }
              frame True {
                n179 = Enqueue Element(queue=w406, element=T2 {"Command"="QUIT", "Configuration"={"Primary Filter"="", "Secondary Filter"="", "Slit Mask"="", "Grating"="", "CS Target"=0.0, "GS Target"=0.0, "Coll Focus"=0, "Camera Focus"=0, "use Flexure Comp?"=FALSE, "WavMode"="", "Slit Toggle"=""}} ("Cluster")) -> ()  [unwired: 2 in, 3 out]
              }
            }
          }
          event Application Instance Close? {
            n180 = event-data() -> ()  [unwired: 1 in, 3 out]
            n181 = Enqueue Element(queue=w408, element=T2 {"Command"="SHUTDOWN", "Configuration"={"Primary Filter"="", "Secondary Filter"="", "Slit Mask"="", "Grating"="", "CS Target"=0.0, "GS Target"=0.0, "Coll Focus"=0, "Camera Focus"=0, "use Flexure Comp?"=FALSE, "WavMode"="", "Slit Toggle"=""}} ("Cluster")) -> ()  [unwired: 2 in, 3 out]
            n182 = event-data() -> ()  [unwired: 2 in, 1 out]
          }
        }
      }
    }
    n183 = Equal?(x=w17, y="SHUTDOWN") -> (x = y?=w28:bool)
    n184 = case shown="Error" w16 {
      tunnel: w15 -> [_ w34]
      frame No Error {
      }
      frame Error {
        n185 = Enqueue Element At Opposite End(queue=w34, element=T2 {"Command"="ERROR", "Configuration"={"Primary Filter"="", "Secondary Filter"="", "Slit Mask"="", "Grating"="", "CS Target"=0.0, "GS Target"=0.0, "Coll Focus"=0, "Camera Focus"=0, "use Flexure Comp?"=FALSE, "WavMode"="", "Slit Toggle"=""}} ("Cluster")) -> ()  [unwired: 2 in, 3 out]
      }
    }
  }
  "error out" <- w4
